vi "GetCollection.vi"(8 "error in (no error)":errorcluster, 10 "collectionName":string="hitran_2012", 11 "MongoDB-Database in":refnum<class "MongoDB-Database.lvclass">) -> (0 "error out":errorcluster, 2 "MongoDB-Collection":refnum<class "MongoDB-Collection.lvclass">, 3 "MongoDB-Database out":refnum<class "MongoDB-Database.lvclass">)   [LabVIEW 2016, in "MongoDB-Database.lvlib" / "MongoDB-Database.lvclass"]
uses:
  MongoDB-Database.lvclass
  D:/Users/blume/Desktop/LV/MongoDB-Driver/MLV DLLs/MongoLabVIEW.dll
  LV/MongoDB-Driver/MLV DLLs/MongoLabVIEW.dll
  MongoDB-Collection/MongoDB-Collection/MongoDB-Collection.lvclass
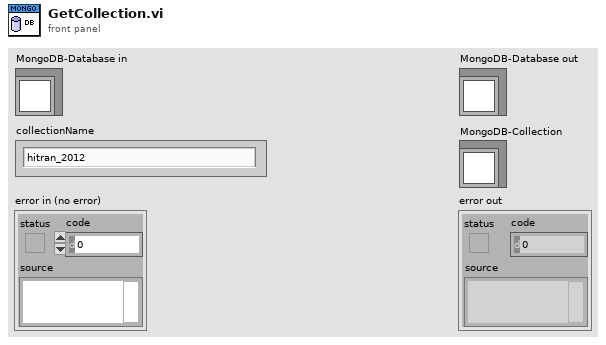
[diagram p1: front panel]
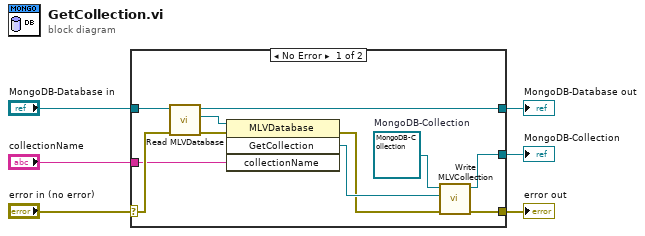
[diagram p0: block diagram]
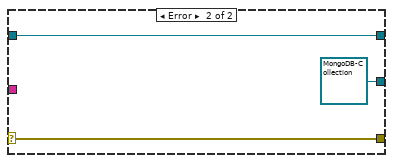
[diagram p2: hidden frame]
diagram:
  n1 = case shown="No Error" "error in (no error)" {
    selector: "error in (no error)" -> [w16 w20]
    tunnel: [w8 w20] -> w5
    tunnel: [w14 w19] -> w3
    tunnel: "MongoDB-Database in" -> [w17 w19]
    tunnel: "collectionName" -> [w12 _]
    tunnel: [w7 refnum<class "MongoDB-Collection.lvclass"> refnum ("MongoDB-Collection out")] -> w1
    frame No Error {
      w11 = refnum<class "MongoDB-Collection.lvclass"> refnum  # MongoDB-Collection
      n2 = call "Read MLVDatabase.vi"("error in (no error)"=w16, "MongoDB-Database in"=w17) -> ("error out"=w13:errorcluster, "MLVDatabase"=w15:refnum<k24>, "MongoDB-Database out"=w14:refnum<class "MongoDB-Database.lvclass">)  [unwired: 7 in]
      n3 = invoke class="MLVDatabase" method="GetCollection"(reference=w15, error in=w13, "collectionName"=w12) -> (error out=w9:errorcluster, "GetCollection"=w10:refnum<k24>)  [unwired: 1 in, 2 out]
      n4 = call "Write MLVCollection.vi"("error in (no error)"=w9, "MLVCollection"=w10, "MongoDB-Collection in"=w11) -> ("error out"=w8:errorcluster, "MongoDB-Collection out"=w7:refnum<class "MongoDB-Collection.lvclass">)  [unwired: 7 in]
    }
    frame Error {
    }
  }
  "error out" <- w5
  "MongoDB-Database out" <- w3
  "MongoDB-Collection" <- w1
